vi "250310_Nikon_Control.vi"() -> ()   [LabVIEW 2025]
doc: "This simple VI control few elements of a Nikon Ti2 microscope.\nAny kind of supplementary element can be controlled with a new event type (flurorescence cube turret for example)"
uses:
  Presets.ctl
panel:
  out "PFS cluster":T1
  in  "Presets":T2=2 items=["1- Bino - Brightfield"=1, "2- Bino - Fluo"=2, "3- Right - Brightfield"=3, "4- Right - Fluo"=4, "5- Left"=5]
  in  "Cluster commandes":T3={"Dia lamp"=TRUE, "Dia lamp intensity"=1689.1304347826087, "Objective"=2, "Light path"=2, "Z pos (µm)"=335593, "Filter wheel 2"=2, "Filter wheel 1"=2, "Shutter 2"=TRUE, "Shutter 1"=TRUE} {"Filter wheel 1" items=["1"=1, "2"=2, "3"=3, "4"=4, "5"=5, "6"=6]; "Filter wheel 2" items=["1"=1, "2"=2, "3"=3, "4"=4, "5"=5, "6"=6]; "Z pos (µm)" min=0 max=990000 step=100 scale=0.0..990000.0; "Light path" items=["1- Eyepiece"=1, "2- Right"=2, "3- Left + Eyepiece"=3, "4- Left"=4]; "Objective" items=["1- PLAN APO 100X 1,45 Oil"=1, "2- Empty"=2, "3- Empty"=3, "4- Empty"=4, "5- Empty"=5, "6- Empty"=6]; "Dia lamp intensity" scale=0.0..2100.0}
  out "Cluster µscope":T4
  in  "stop":bool
  in  "NikonTi2AxLib.INikonTi2AxMicroscope":refnum<k7>
  out "error out":errorcluster={"status"=TRUE, "code"=-9, "source"="Exception occured in Nikon.Ti2.Microscope.1: Failed in 231026_NikonTi2_Indicators_v2.vi"} caption="sortie d'erreur"
  in  "error in":errorcluster caption="entrée d'erreur"
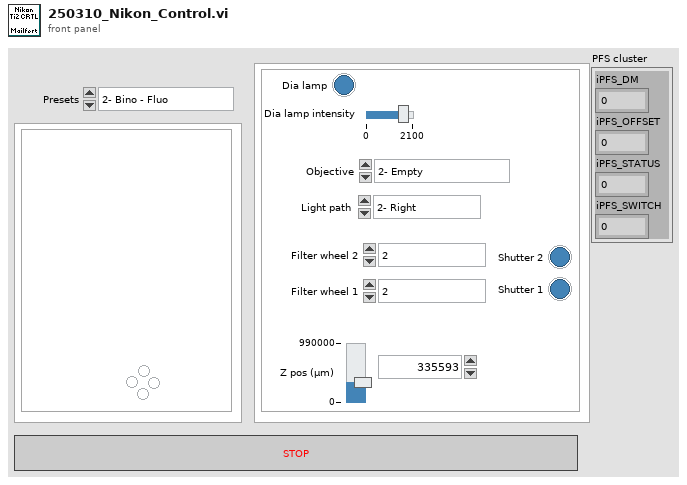
[diagram p1: front panel]
types:
  T1 = cluster{"iPFS_DM":i32, "iPFS_OFFSET":i32, "iPFS_STATUS":i32, "iPFS_SWITCH":i32}
  T2 = typedef "Presets.ctl" = u8
  T3 = cluster{"Dia lamp":bool, "Dia lamp intensity":dbl, "Objective":i32, "Light path":u32, "Z pos (µm)":i32, "Filter wheel 2":u32, "Filter wheel 1":u32, "Shutter 2":bool, "Shutter 1":bool}
  T4 = cluster{"Eyepiece":bool, "Right":bool, "Left + Eyepiece":bool, "Left":bool}
  T5 = cluster{"iNOSEPIECE":i32, "iLIGHTPATH":i32, "iDIA_LAMP_Switch":i32, "iDIA_LAMP_Pos":i32, "iZPOSITION":i32, "iPFS_SWITCH":i32, "iPFS_STATUS":i32, "iPFS_OFFSET":i32, "iTURRET2POS":i32, "Value":i32, "iTURRET1POS":i32, "Value":i32, "iOPTZOOM":i32}
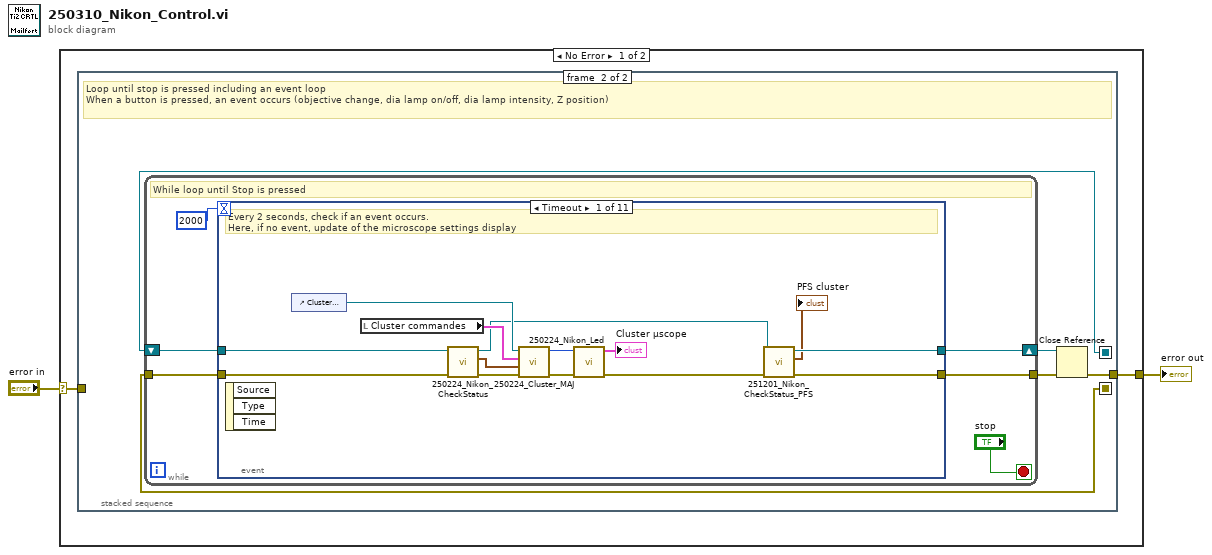
[diagram p0: block diagram]
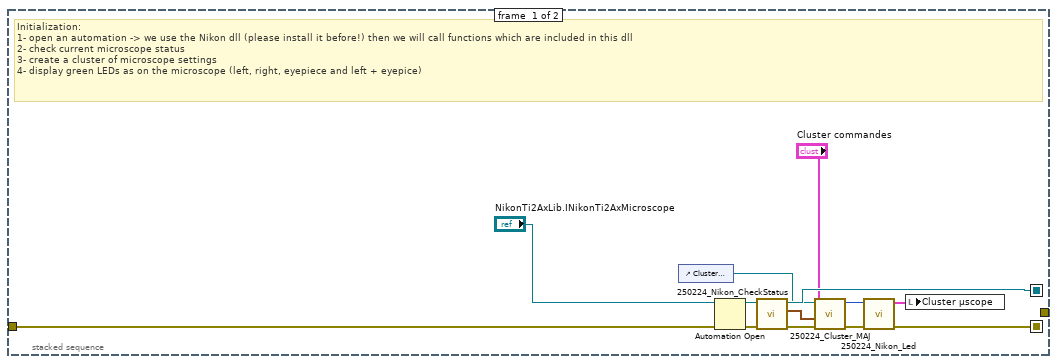
[diagram p2: hidden frame]
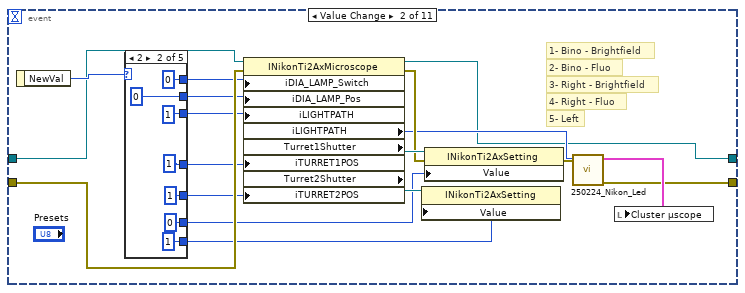
[diagram p3: hidden frame]
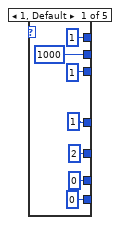
[diagram p4: hidden frame]
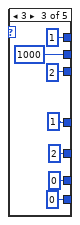
[diagram p5: hidden frame]
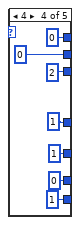
[diagram p6: hidden frame]
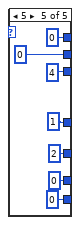
[diagram p7: hidden frame]
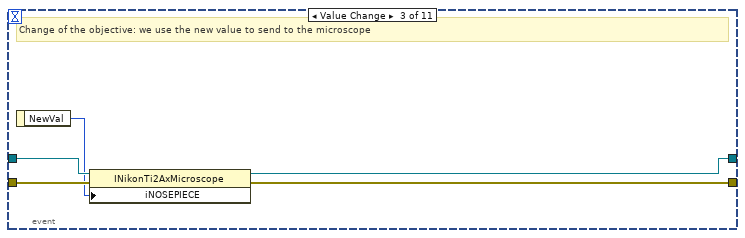
[diagram p8: hidden frame]
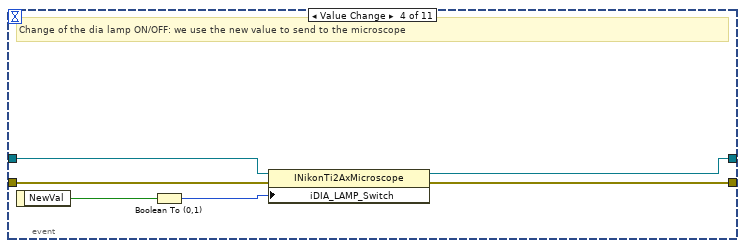
[diagram p9: hidden frame]
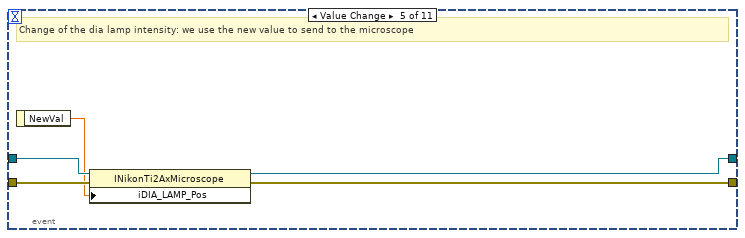
[diagram p10: hidden frame]
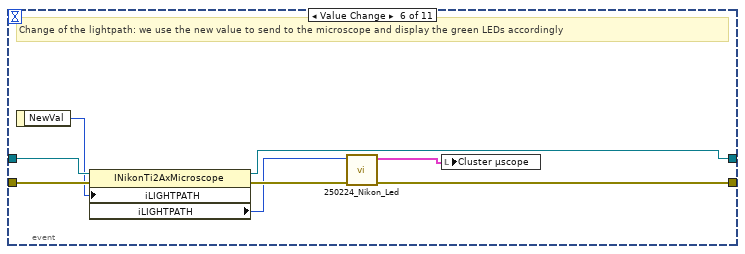
[diagram p11: hidden frame]
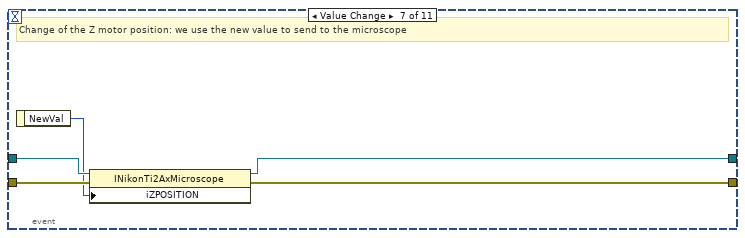
[diagram p12: hidden frame]
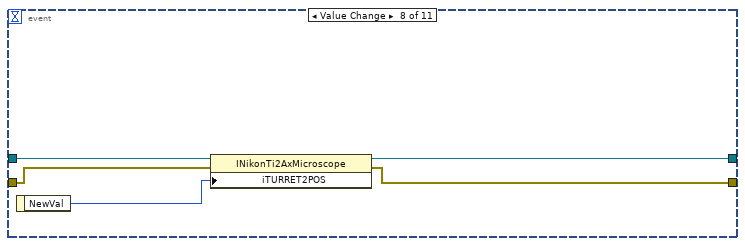
[diagram p13: hidden frame]
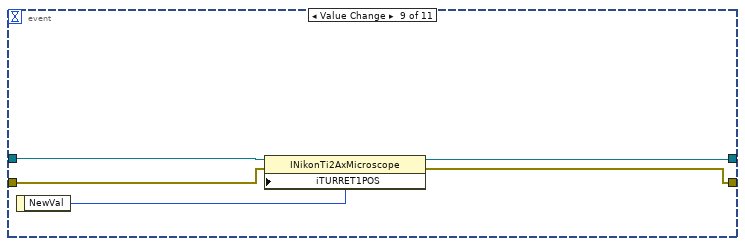
[diagram p14: hidden frame]
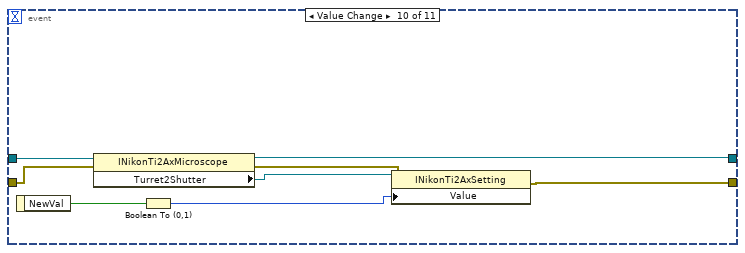
[diagram p15: hidden frame]
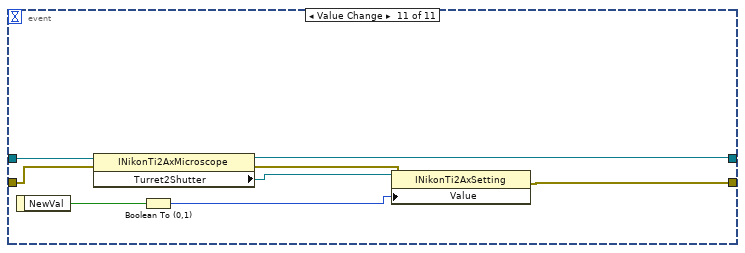
[diagram p16: hidden frame]
diagram:
  n1 = case shown="No Error" "error in" {
    selector: "error in" -> [w4 w151]
    tunnel: [w3 w151] -> w1
    frame No Error {
      n2 = stacked-sequence {
        seq-local: [w13 _] -> [_ w22]
        seq-local: [w7 _] -> [_ w18]
        tunnel: w4 -> [w14 _]
        tunnel: [_ w19] -> w3
        frame #0 {
          # "Initialization:\n1- open an automation -> we use the Nikon dll (please install it before!) then we will call functions which are included in this dll\n2- check current microscope status\n3- create a cluster of microscope settings\n4- display green LEDs as on the microscope (left, right, eyepiece and left + eyepice)"
          n3 = control-ref of="Cluster commandes"() -> (w6:refnum<vi>)
          n4 = Automation Open(error in (no error)=w14, Automation Refnum="NikonTi2AxLib.INikonTi2AxMicroscope") -> (Automation Refnum=w16:refnum<k7>, error out=w15:errorcluster)  [unwired: 2 in]
          n5 = call "250224_Nikon_CheckStatus.vi"("error in"=w15, "NikonTi2AxLib.INikonTi2AxMicroscope"=w16) -> ("error out"=w9:errorcluster, "Nikon Cluster"=w12:T5, "reference out"=w13:refnum<k7>)  [unwired: 7 in]
          n6 = call "250224_Cluster_MAJ.vi"("error in (no error)"=w9, "Nikon Cluster"=w12, 10:"Cluster commandes"="Cluster commandes", 11:"Cluster commandes"=w6) -> ("error out"=w8:errorcluster, "iLIGHTPATH"=w10:i32)  [unwired: 6 in]
          n7 = call "250224_Nikon_Led.vi"("error in"=w8, "Light path"=w10) -> ("error out"=w7:errorcluster, "Cluster µscope"=w11:T4)  [unwired: 8 in]
          n8 = local write "Cluster µscope"(w11) -> ()
        }
        frame #1 {
          # "Loop until stop is pressed including an event loop\nWhen a button is pressed, an event occurs (objective change, dia lamp on/off, dia lamp intensity, Z position)"
          n9 = while {
            shift-right: [w24] -> w21
            shift-left: w22 -> [w25]
            tunnel: w18 -> [w28]
            tunnel: [w23] -> w20
            stop <- "stop" stop-if-true
            # "While loop until Stop is pressed"
            n10 = event shown="[0] Timeout" {
              selector: _ -> [_ _ _ _ _ _ _ _ _ _ _]
              dyn-events: _ -> [_ _ _ _ _ _ _ _ _ _ _]
              timeout: 2000 -> [_ _ _ _ _ _ _ _ _ _ _]
              tunnel: [w33 w59 w97 w103 w108 w116 w122 w126 w130 w137 w145] -> w23
              tunnel: w28 -> [w42 w54 w99 w105 w110 w117 w123 w127 w133 w142 w150]
              tunnel: w25 -> [w41 w55 w100 w106 w111 w118 w124 w129 w134 w141 w149]
              tunnel: [w31 w43 w98 w104 w109 w119 w120 w125 w131 w138 w146] -> w24
              event Timeout {
                # "Every 2 seconds, check if an event occurs.\nHere, if no event, update of the microscope settings display"
                n11 = event-data() -> ()  [unwired: 1 in, 3 out]
                n12 = control-ref of="Cluster commandes"() -> (w35:refnum<vi>)
                n13 = local read "Cluster commandes"() -> (w36:T3)
                n14 = call "250224_Nikon_CheckStatus.vi"("error in"=w42, "NikonTi2AxLib.INikonTi2AxMicroscope"=w41) -> ("error out"=w39:errorcluster, "Nikon Cluster"=w29:T5, "reference out"=w32:refnum<k7>)  [unwired: 7 in]
                n15 = call "250224_Cluster_MAJ.vi"("error in (no error)"=w39, "Nikon Cluster"=w29, 10:"Cluster commandes"=w36, 11:"Cluster commandes"=w35) -> ("error out"=w38:errorcluster, "iLIGHTPATH"=w37:i32)  [unwired: 6 in]
                n16 = call "250224_Nikon_Led.vi"("error in"=w38, "Light path"=w37) -> ("error out"=w34:errorcluster, "Cluster µscope"=→"Cluster µscope":T4)  [unwired: 8 in]
                n17 = call "251201_Nikon_CheckStatus_PFS.vi"("error in"=w34, "NikonTi2AxLib.INikonTi2AxMicroscope"=w32) -> ("error out"=w33:errorcluster, "PFS cluster"=→"PFS cluster":T1, "reference out"=w31:refnum<k7>)  [unwired: 7 in]
              }
              event Value Change {
                # "1- Bino - Brightfield"
                # "5- Left"
                # "4- Right - Fluo"
                # "3- Right - Brightfield"
                # "2- Bino - Fluo"
                n18 = event-data() -> ("NewVal"=w58:T2)  [unwired: 1 in]
                n19 = case shown="2" w58 {
                  tunnel: [1 0 1 0 0] -> w50
                  tunnel: [1000 0 1000 0 0] -> w49
                  tunnel: [1 ("iLIGHTPATH") 1 ("iLIGHTPATH") 2 ("iLIGHTPATH") 2 ("iLIGHTPATH") 4 ("iLIGHTPATH")] -> w48
                  tunnel: [1 ("iLIGHTPATH") 1 ("iLIGHTPATH") 1 ("iLIGHTPATH") 1 ("iLIGHTPATH") 1 ("iLIGHTPATH")] -> w47
                  tunnel: [2 ("iLIGHTPATH") 1 ("iLIGHTPATH") 2 ("iLIGHTPATH") 1 ("iLIGHTPATH") 2 ("iLIGHTPATH")] -> w46
                  tunnel: [0 ("iLIGHTPATH") 0 ("iLIGHTPATH") 0 ("iLIGHTPATH") 0 ("iLIGHTPATH") 0 ("iLIGHTPATH")] -> w45
                  tunnel: [0 ("iLIGHTPATH") 1 ("iLIGHTPATH") 0 ("iLIGHTPATH") 1 ("iLIGHTPATH") 0 ("iLIGHTPATH")] -> w44
                  frame 1, Default {
                  }
                  frame 2 {
                  }
                  frame 3 {
                  }
                  frame 4 {
                  }
                  frame 5 {
                  }
                }
                n20 = property class="INikonTi2AxMicroscope"(reference=w55, error in=w54, "iDIA_LAMP_Switch"=w50, "iDIA_LAMP_Pos"=w49, "iLIGHTPATH"=w48, "iTURRET1POS"=w47, "iTURRET2POS"=w46) -> (reference out=w43:refnum<k7>, error out=w53:errorcluster, "iLIGHTPATH"=w51:i32, "Turret1Shutter"=w57:refnum<k7>, "Turret2Shutter"=w56:refnum<k7>)
                n21 = property class="INikonTi2AxSetting"(reference=w56, "Value"=w44) -> ()  [unwired: 1 in, 2 out]
                n22 = property class="INikonTi2AxSetting"(reference=w57, error in=w53, "Value"=w45) -> (error out=w52:errorcluster)  [unwired: 1 out]
                n23 = call "250224_Nikon_Led.vi"("error in"=w52, "Light path"=w51) -> ("error out"=w59:errorcluster, "Cluster µscope"=w60:T4)  [unwired: 8 in]
                n24 = local write "Cluster µscope"(w60) -> ()
              }
              event "Cluster commandes.Objective": Value Change {
                # "Change of the objective: we use the new value to send to the microscope"
                n25 = event-data() -> ("NewVal"=w96:i32)  [unwired: 1 in]
                n26 = property class="INikonTi2AxMicroscope"(reference=w100, error in=w99, "iNOSEPIECE"=w96) -> (reference out=w98:refnum<k7>, error out=w97:errorcluster)
              }
              event "Cluster commandes.Dia lamp": Value Change {
                # "Change of the dia lamp ON/OFF: we use the new value to send to the microscope"
                n27 = event-data() -> ("NewVal"=w102:bool)  [unwired: 1 in]
                n28 = Boolean To (0,1)(Boolean=w102) -> (0, 1=w101:i16)
                n29 = property class="INikonTi2AxMicroscope"(reference=w106, error in=w105, "iDIA_LAMP_Switch"=w101) -> (reference out=w104:refnum<k7>, error out=w103:errorcluster)
              }
              event "Cluster commandes.Dia lamp intensity": Value Change {
                # "Change of the dia lamp intensity: we use the new value to send to the microscope"
                n30 = event-data() -> ("NewVal"=w107:dbl)  [unwired: 1 in]
                n31 = property class="INikonTi2AxMicroscope"(reference=w111, error in=w110, "iDIA_LAMP_Pos"=w107) -> (reference out=w109:refnum<k7>, error out=w108:errorcluster)
              }
              event "Cluster commandes.Light path": Value Change {
                # "Change of the lightpath: we use the new value to send to the microscope and display the green LEDs accordingly"
                n32 = event-data() -> ("NewVal"=w113:u32)  [unwired: 1 in]
                n33 = property class="INikonTi2AxMicroscope"(reference=w118, error in=w117, "iLIGHTPATH"=w113) -> (reference out=w119:refnum<k7>, error out=w115:errorcluster, "iLIGHTPATH"=w114:i32)
                n34 = call "250224_Nikon_Led.vi"("error in"=w115, "Light path"=w114) -> ("error out"=w116:errorcluster, "Cluster µscope"=w112:T4)  [unwired: 8 in]
                n35 = local write "Cluster µscope"(w112) -> ()
              }
              event "Cluster commandes.Z pos (µm)": Value Change {
                # "Change of the Z motor position: we use the new value to send to the microscope"
                n36 = event-data() -> ("NewVal"=w121:i32)  [unwired: 1 in]
                n37 = property class="INikonTi2AxMicroscope"(reference=w124, error in=w123, "iZPOSITION"=w121) -> (reference out=w120:refnum<k7>, error out=w122:errorcluster)
              }
              event "Cluster commandes.Filter wheel 2": Value Change {
                n38 = event-data() -> ("NewVal"=w128:u32)  [unwired: 1 in]
                n39 = property class="INikonTi2AxMicroscope"(reference=w129, error in=w127, "iTURRET2POS"=w128) -> (reference out=w125:refnum<k7>, error out=w126:errorcluster)
              }
              event "Cluster commandes.Filter wheel 1": Value Change {
                n40 = event-data() -> ("NewVal"=w132:u32)  [unwired: 1 in]
                n41 = property class="INikonTi2AxMicroscope"(reference=w134, error in=w133, "iTURRET1POS"=w132) -> (reference out=w131:refnum<k7>, error out=w130:errorcluster)
              }
              event "Cluster commandes.Shutter 2": Value Change {
                n42 = event-data() -> ("NewVal"=w136:bool)  [unwired: 1 in]
                n43 = property class="INikonTi2AxMicroscope"(reference=w141, error in=w142) -> (reference out=w138:refnum<k7>, error out=w139:errorcluster, "Turret2Shutter"=w140:refnum<k7>)
                n44 = Boolean To (0,1)(Boolean=w136) -> (0, 1=w135:i16)
                n45 = property class="INikonTi2AxSetting"(reference=w140, error in=w139, "Value"=w135) -> (error out=w137:errorcluster)  [unwired: 1 out]
              }
              event "Cluster commandes.Shutter 1": Value Change {
                n46 = event-data() -> ("NewVal"=w144:bool)  [unwired: 1 in]
                n47 = property class="INikonTi2AxMicroscope"(reference=w149, error in=w150) -> (reference out=w146:refnum<k7>, error out=w147:errorcluster, "Turret2Shutter"=w148:refnum<k7>)
                n48 = Boolean To (0,1)(Boolean=w144) -> (0, 1=w143:i16)
                n49 = property class="INikonTi2AxSetting"(reference=w148, error in=w147, "Value"=w143) -> (error out=w145:errorcluster)  [unwired: 1 out]
              }
            }
          }
          n50 = Close Reference(reference=w21, error in (no error)=w20) -> (error out=w19:errorcluster)
        }
      }
    }
    frame Error {
    }
  }
  "error out" <- w1
